vi "eGateHSP_InitBuffer.vi"(7 "path in":path, 8 "Fehler (Eingang, kein Fehler)":errorcluster, 9 "bufferIndex":i32, 11 "e.gate Configuration":T1 {"StartTime" format="%#.10f"; "dActTimeToSecondFactor" format="%#.10f"; "StartTimeToDayFactor" format="%#_10f"}) -> (0 "Fehler (Ausgang)":errorcluster, 3 "e.gate Configuration 2":T1 {"StartTime" format="%#.10f"; "dActTimeToSecondFactor" format="%#.10f"; "StartTimeToDayFactor" format="%#_10f"})   [LabVIEW 2016]
uses:
  e.gate Configuration.ctl
  e.gate Channel Data.ctl
  e.gate Data Type.ctl
  e.gate Protocol Type.ctl
  e.gate Module  Data.ctl
  e.gateHSP_DLLhandle.ctl
panel:
  out "Rückgabewert":i32
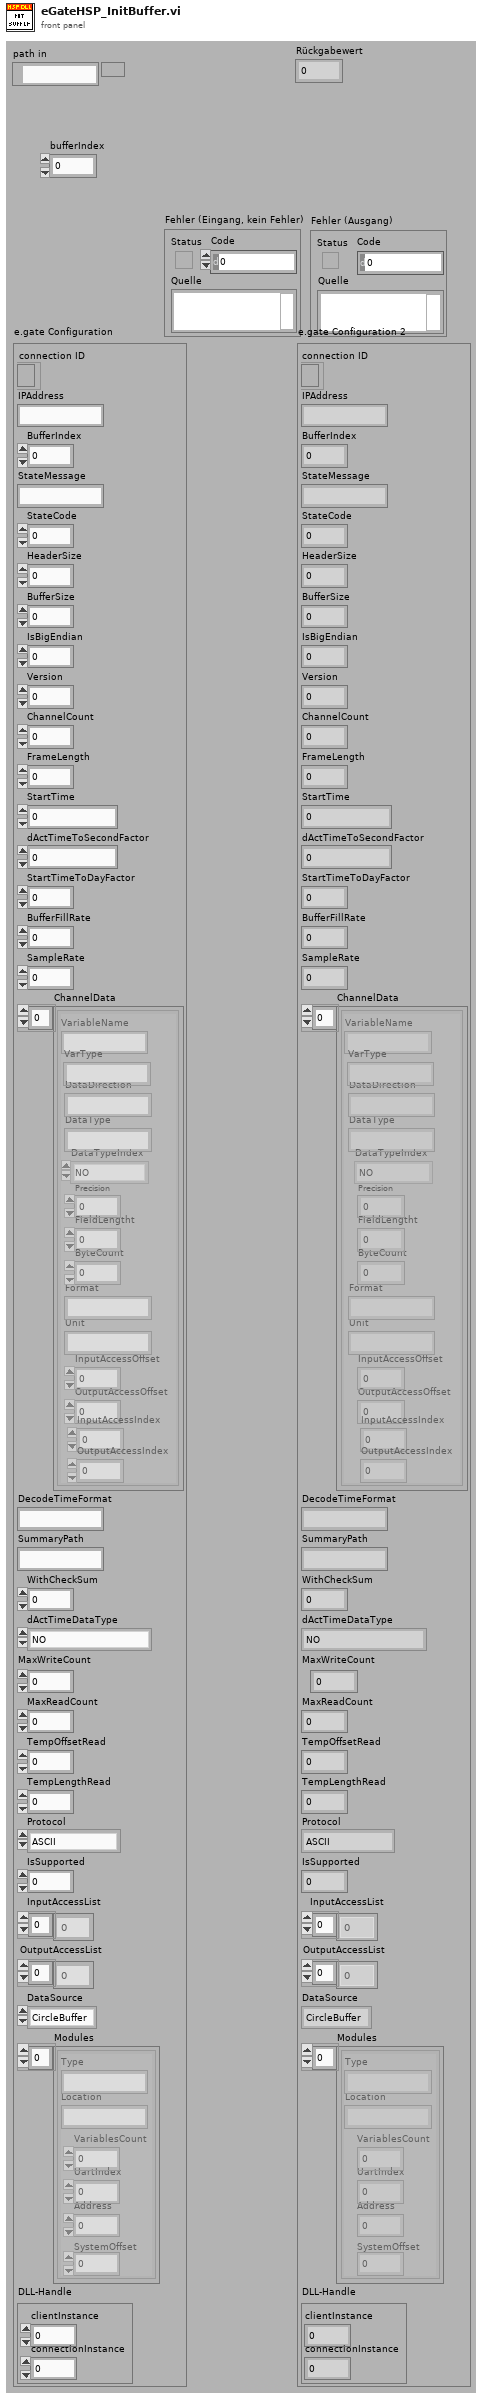
[diagram p1: front panel]
types:
  T1 = typedef "e.gate Configuration.ctl" = cluster{"connection ID":refnum<k5>, "IPAddress":string, "BufferIndex":i32, "StateMessage":string, "StateCode":i8, "HeaderSize":i32, "BufferSize":i32, "IsBigEndian":i32, "Version":i32, "ChannelCount":i32, "FrameLength":i32, "StartTime":dbl, "dActTimeToSecondFactor":dbl, "StartTimeToDayFactor":dbl, "BufferFillRate":dbl, "SampleRate":dbl, "ChannelData":T2[], "DecodeTimeFormat":string, "SummaryPath":string, "WithCheckSum":i32, "dActTimeDataType":T3, "MaxWriteCount":i32, "MaxReadCount":i32, "TempOffsetRead":i32, "TempLengthRead":i32, "Protocol":T4, "IsSupported":i32, "InputAccessList":i32[], "OutputAccessList":i32[], "DataSource":enum16{"CircleBuffer", "test.con Logger", "test.con Archive"}, "Modules":T5[], "DLL-Handle":T6}
  T2 = typedef "e.gate Channel Data.ctl" = cluster{"VariableName":string, "DataDirection":string, "DataType":string, "DataTypeIndex":T3, "Precision":i16, "FieldLengtht":i16, "ByteCount":i32, "Format":string, "Unit":string, "InputAccessOffset":i32, "OutputAccessOffset":i16, "InputAccessIndex":i16, "OutputAccessIndex":i16, "VarType":string}
  T3 = typedef "e.gate Data Type.ctl" = enum16{"NO", "BOOL", "SINT8", "USINT8", "SINT16", "USINT16", "SINT32", "USINT32", "FLOAT", "SET8", "SET16", "SET32", "DOUBLE", "SINT64", "USINT64", "SET64"}
  T4 = typedef "e.gate Protocol Type.ctl" = enum16{"ASCII", "HighspeedPort Online", "HighspeedPort Buffer", "eGateHighspeedPortDLL "}
  T5 = typedef "e.gate Module  Data.ctl" = cluster{"Type":string, "Location":string, "VariablesCount":i16, "UartIndex":i16, "Address":i16, "SystemOffset":i16}
  T6 = typedef "e.gateHSP_DLLhandle.ctl" = cluster{"clientInstance":i32, "connectionInstance":i32}
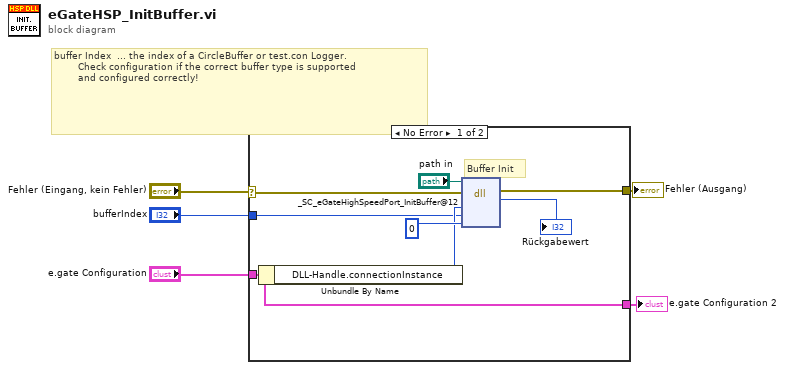
[diagram p0: block diagram]
diagram:
  # "buffer Index\t\t... the index of a CircleBuffer or test.con Logger.\n\t\t\t\t\t\t\t\tCheck configuration if the correct buffer type is supported\n\t\t\t\t\t\t\t\tand configured correctly!"
  n1 = case shown="No Error" "Fehler (Eingang, kein Fehler)" {
    selector: "Fehler (Eingang, kein Fehler)" -> [w12 w14]
    tunnel: [w11 w14] -> w4
    tunnel: "bufferIndex" -> [w8 _]
    tunnel: "e.gate Configuration" -> [w10 _]
    tunnel: [w10 _] -> w1
    frame No Error {
      # "Buffer Init"
      n2 = Unbundle By Name(w10) -> ("DLL-Handle.connectionInstance"=w9:i32)
      n3 = dll-call lib="eGateHighSpeedPort.dll" fn="_SC_eGateHighSpeedPort_InitBuffer@12"(path in="path in", error in=w12, "connectionInstance"=w9, "bufferIndex"=w8, "autoRun"=0) -> (error out=w11:errorcluster, "Rückgabewert"=→"Rückgabewert":i32)  [unwired: 4 in, 1 out]
    }
    frame Error {
    }
  }
  "Fehler (Ausgang)" <- w4
  "e.gate Configuration 2" <- w1
